vi "zad2.vi"() -> ()   [LabVIEW 2018]
uses:
  System.Management
panel:
  out "Array 2":string[](array[string])
  in  "stop":bool
  out "Waveform Chart":dbl(graph)
  out "Array":string[](array[string])
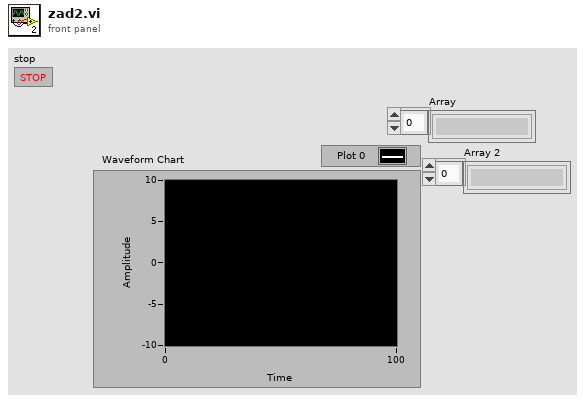
[diagram p1: front panel]
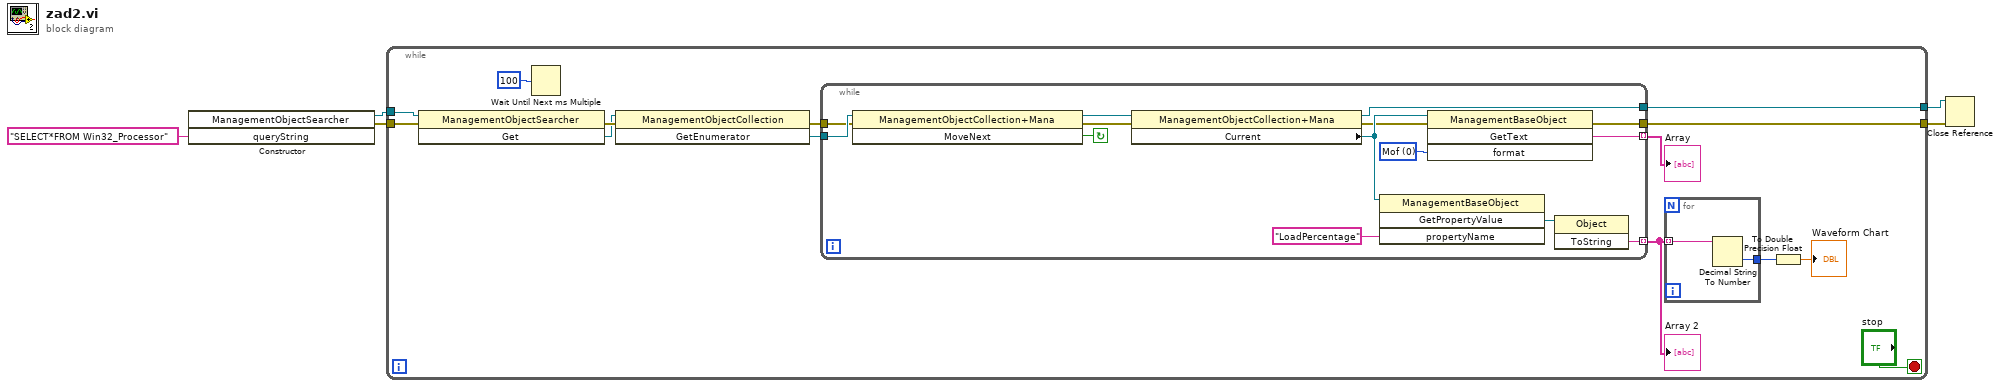
[diagram p0: block diagram]
diagram:
  n1 = constructor class="ManagementObjectSearcher"("queryString"="SELECT*FROM Win32_Processor") -> (reference out=w4:refnum<k24>, error out=w3:errorcluster)  [unwired: 3 in, 2 out]
  n2 = while {
    tunnel: w4 -> [w16]
    tunnel: w3 -> [w15]
    tunnel: [w7] -> w2
    tunnel: [w6] -> w1
    stop <- "stop" stop-if-true
    n3 = invoke class="ManagementObjectSearcher" method="Get"(reference=w16, error in=w15) -> (error out=w14:errorcluster, "Get"=w13:refnum<k24>)  [unwired: 1 in, 1 out]
    n4 = Wait Until Next ms Multiple(millisecond multiple=u32 100) -> ()  [unwired: 1 out]
    n5 = invoke class="ManagementObjectCollection" method="GetEnumerator"(reference=w13, error in=w14) -> (error out=w18:errorcluster, "GetEnumerator"=w19:refnum<k24>)  [unwired: 1 in, 1 out]
    n6 = while {
      tunnel: w19 -> [w35]
      tunnel: w18 -> [w33]
      tunnel: [w29] -> w17 mode=indexing
      tunnel: [w25] -> w10 mode=indexing
      tunnel: [w23] -> w7
      tunnel: [w22] -> w6
      stop <- w34 continue-if-true
      w30 = 0 items=["Mof", "CimDtd20", "WmiDtd20"] ("format")
      n7 = invoke class="ManagementObjectCollection+Mana" method="MoveNext"(reference=w35, error in=w33) -> (reference out=w31:refnum<k24>, error out=w32:errorcluster, "MoveNext"=w34:bool)  [unwired: 1 in]
      n8 = property class="ManagementObjectCollection+Mana"(reference=w31, error in=w32) -> (reference out=w23:refnum<k24>, error out=w24:errorcluster, "Current"=w28:refnum<k24>)
      n9 = invoke class="ManagementBaseObject" method="GetPropertyValue"(reference=w28, "propertyName"="LoadPercentage") -> ("GetPropertyValue"=w26:refnum<k24>)  [unwired: 2 in, 3 out]
      n10 = invoke class="ManagementBaseObject" method="GetText"(reference=w28, error in=w24, "format"=w30) -> (error out=w22:errorcluster, "GetText"=w29:string)  [unwired: 1 in, 2 out]
      n11 = invoke class="Object" method="ToString"(reference=w26) -> ("ToString"=w25:string)  [unwired: 2 in, 2 out]
    }
    "Array" <- w17
    "Array 2" <- w10
    n12 = for {
      tunnel: w10 -> [w21] mode=indexing
      tunnel: [w20] -> w9
      n13 = Decimal String To Number(string=w21) -> (number=w20:i32)  [unwired: 2 in, 1 out]
    }
    n14 = To Double Precision Float(number=w9) -> (double precision float=→"Waveform Chart":dbl)
  }
  n15 = Close Reference(reference=w2, error in (no error)=w1) -> ()  [unwired: 1 out]
